vi "SpectrumRaw.vi"(7 "Type":T1, 8 "error in (no error)":errorcluster, 11 "Instruments in":refnum<class "Instruments.lvclass">) -> (0 "error out":errorcluster, 2 "Peak Wl":dbl, 3 "Instruments out":refnum<class "Instruments.lvclass">, 4 "Remeasure":bool, 5 "Saturated?":bool)   [LabVIEW 2012, in "Instruments.lvclass"]
uses:
  Instruments.lvclass
  Controls/SpectrometerOphirSelector.ctl
  Instruments.lvclass/Instruments.ctl
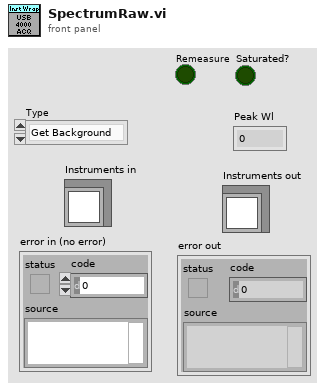
[diagram p1: front panel]
types:
  T1 = typedef "SpectrometerOphirSelector.ctl" = enum16{"Get Background", "Measure", "Measure50", "Raw"}
  T2 = typedef "USB4000_Data.ctl" = cluster{"Wrapper Out":u32, "Number of Spectrometers":i32, "Wavelength":dbl[], "EL Spectrum":dbl[], "Int Time (usec)":i32, bool, "Background":dbl[]}
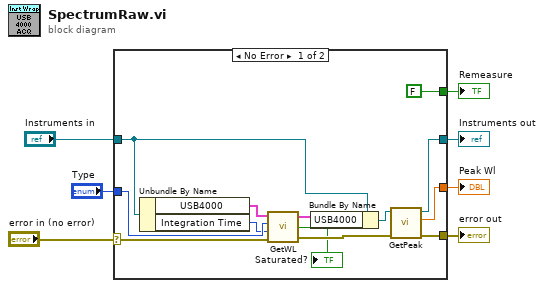
[diagram p0: block diagram]
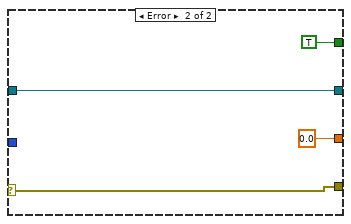
[diagram p2: hidden frame]
diagram:
  n1 = case shown="No Error" "error in (no error)" {
    selector: "error in (no error)" -> [w17 w24]
    tunnel: [w10 w24] -> w6
    tunnel: [w12 w23] -> w4
    tunnel: "Instruments in" -> [w15 w23]
    tunnel: "Type" -> [w19 _]
    tunnel: [FALSE TRUE] -> w2
    tunnel: [w11 0.0 ("Peak Wl")] -> w1
    frame No Error {
      n2 = Unbundle By Name(w15) -> ("USB4000"=w16:T2, "Integration Time"=w18:i32)
      n3 = call "GetWL.vi"("error in (no error)"=w17, "Integration Time"=w18, "Type"=w19, "USB4000 Params In"=w16) -> ("error out"=w9:errorcluster, "Saturated?"=→"Saturated?":bool, "USB4000 Params Out"=w14:T2)
      n4 = Bundle By Name(cluster=w15, "USB4000"=w14) -> (w13:refnum<class "Instruments.lvclass">)
      n5 = call-dynamic "GetPeak.vi"("error in (no error)"=w9, "Instruments in"=w13) -> ("error out"=w10:errorcluster, "Peak Wl"=w11:dbl, "Instruments out"=w12:refnum<class "Instruments.lvclass">)  [unwired: 7 in]
    }
    frame Error {
    }
  }
  "error out" <- w6
  "Instruments out" <- w4
  "Peak Wl" <- w1
  "Remeasure" <- w2
